vi "UI-Set Maximize Button Value.vi"(8 "Error In":errorcluster, 10 "Value (F)":bool, 11 "Appearance Actor in":refnum<class "Appearance Actor.lvclass">) -> (0 "Error Out":errorcluster, 3 "Appearance Actor out":refnum<class "Appearance Actor.lvclass">)   [LabVIEW 2021, in "Appearance Actor.lvlib" / "Appearance Actor.lvclass"]
uses:
  Appearance Actor.lvclass
  Appearance Actor.lvclass/Appearance Actor.ctl
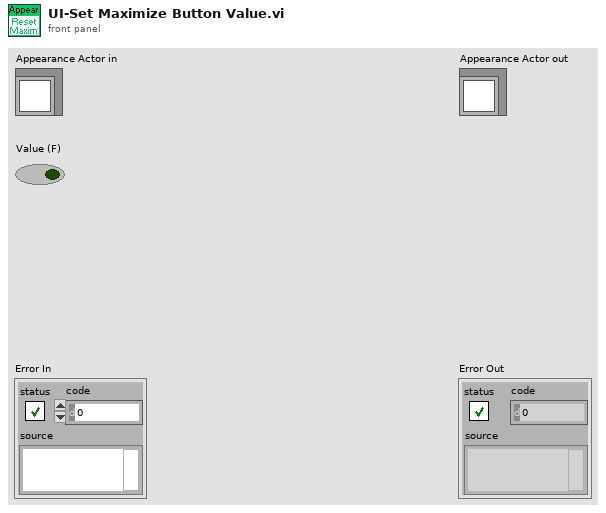
[diagram p1: front panel]
types:
  T1 = typedef "Appearance Actor.lvlib/Appearance Actor.lvclass/UI Controls--map.ctl" = map{string, T2}
  T2 = typedef "Appearance Actor.lvlib/Appearance Actor.lvclass/Element Controls--map.ctl" = map{string, T3}
  T3 = typedef "Appearance Actor.lvlib/Appearance Actor.lvclass/Controls--map.ctl" = map{string, refnum<vi>}
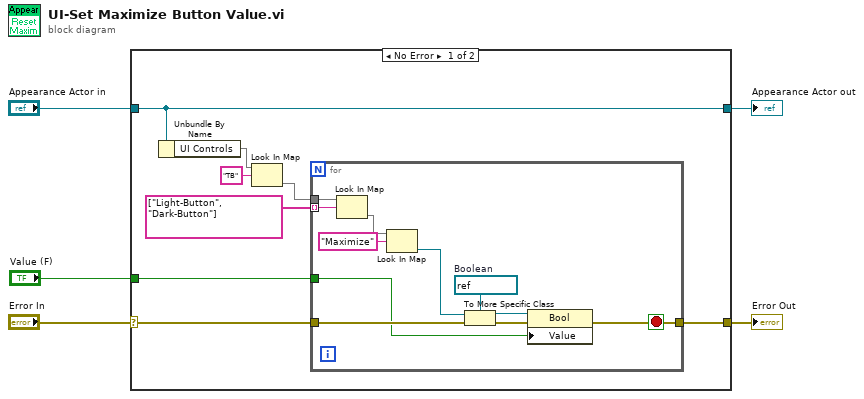
[diagram p0: block diagram]
diagram:
  n1 = case shown="No Error" "Error In" {
    selector: "Error In" -> [w8 w26]
    tunnel: [w7 w26] -> w4
    tunnel: [w13 w25] -> w2
    tunnel: "Appearance Actor in" -> [w13 w25]
    tunnel: "Value (F)" -> [w6 _]
    frame No Error {
      n2 = Unbundle By Name(w13) -> ("UI Controls"=w12:T1)
      n3 = Look In Map(map=w12, key="TB") -> (value=w10:T2)  [unwired: 1 in, 1 out]
      n4 = for {
        tunnel: w10 -> [w24]
        tunnel: string[] ["Light-Button", "Dark-Button"] ("key") -> [w23] mode=indexing
        tunnel: w8 -> [w17]
        tunnel: [w16] -> w7
        tunnel: w6 -> [w14]
        stop <- w16 stop-if-true
        w18 = refnum<vi> refnum  # Boolean
        n5 = Look In Map(map=w24, key=w23) -> (value=w22:T3)  [unwired: 1 in, 1 out]
        n6 = Look In Map(map=w22, key="Maximize") -> (value=w15:refnum<vi>)  [unwired: 1 in, 1 out]
        n7 = To More Specific Class(target class=w18, reference=w15, error in=w17) -> (specific class reference=w19:refnum<vi>, error out=w20:errorcluster)
        n8 = property class="Bool"(reference=w19, error in=w20, "Value"=w14) -> (error out=w16:errorcluster)  [unwired: 1 out]
      }
    }
    frame Error {
    }
  }
  "Error Out" <- w4
  "Appearance Actor out" <- w2
